vi "Get All.vi"(0 "Tree Reference In":refnum<vi>, 2 "Starting Tag":string, 3 "Input Tree Items(DO NOT WIRE)":string[](array[string]), 5 "error in (no error)":errorcluster) -> (14 "Tree Reference Out":refnum<vi>, 16 "Current Item":string, 17 "Output Tree Items":string[](array[string]), 19 "error out":errorcluster)   [LabVIEW 2011, in "VITesterUtilities.lvlib"]
doc: "Retrieves all elements in tree at and below the starting tag. When Starting Tag and Input Tree Items are left unwired it will return all elements in the tree."
uses:
  Libraries/VITesterUtilities.lvlib
panel:
  in  "Identical VI Refnum":refnum<vi>
  # "VI LOCALS"
  # "VI OUTPUTS"
  # "VI INPUTS"
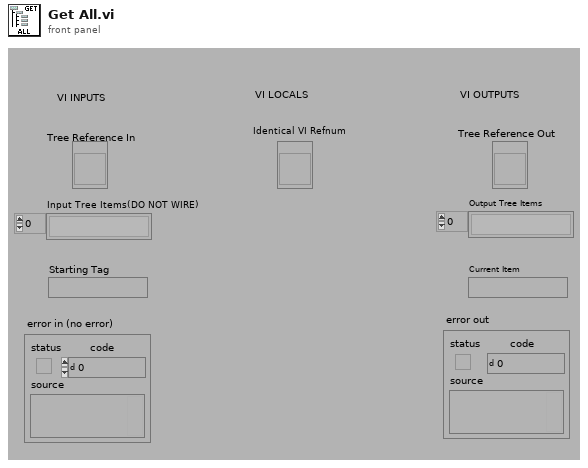
[diagram p1: front panel]
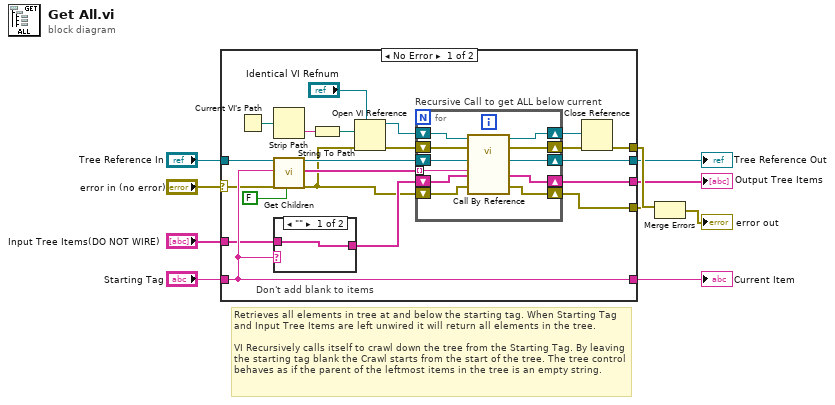
[diagram p0: block diagram]
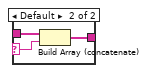
[diagram p2: hidden frame]
diagram:
  # "Retrieves all elements in tree at and below the starting tag. When Starting Tag and Input Tree Items are left unwired it will return all elements in the tree. \n\nVI Recursively calls itself to crawl down the tree from the Starting Tag. By leaving the starting tag blank the Crawl starts from the start of the tree. The tree control behaves as if the parent of the leftmost items in the tree is an empty string."
  n1 = case shown="No Error" "error in (no error)" {
    selector: "error in (no error)" -> [w12 w47]
    tunnel: "Tree Reference In" -> [w31 w48]
    tunnel: [w30 w48] -> w6
    tunnel: "Starting Tag" -> [w29 w50]
    tunnel: [w28 w49] -> w4
    tunnel: [w29 w50] -> w3
    tunnel: "Input Tree Items(DO NOT WIRE)" -> [w27 w49]
    tunnel: [w26 w47] -> w10
    tunnel: [w25 w47] -> w9
    frame No Error {
      n2 = Current VI's Path() -> (path=w17:path)
      n3 = Strip Path(path=w17) -> (name=w15:string)  [unwired: 1 out]
      n4 = call "Get Children.vi"("Tree Reference In"=w31, "Parent Tag"=w29, "error in (no error)"=w12, "Use Current"=FALSE) -> ("Tree Reference Out"=w24:refnum<vi>, "Children Tags"=w20:string[], "error out"=w11:errorcluster)  [unwired: 13 in]
      n5 = case "Don't add blank to items" shown="\"\"" w29 {
        selector: w29 -> [_ w33]
        tunnel: w27 -> [w32 w35]
        tunnel: [w32 w34] -> w19
        frame "" {
        }
        frame Default {
          n6 = Build Array (concatenate)(w35, w33) -> (w34:string[])
        }
      }
      n7 = String To Path(string=w15) -> (path=w16:path)
      n8 = Open VI Reference(type specifier VI Refnum (for type only)="Identical VI Refnum", vi path=w16, error in (no error)=w11) -> (vi reference=w18:refnum<vi>, error out=w22:errorcluster)  [unwired: 3 in]
      n9 = for "Recursive Call to get ALL below current" {
        shift-right: [w44] -> w25
        shift-left: w11 -> [w45]
        shift-right: [w43] -> w30
        shift-left: w24 -> [w46]
        shift-right: [w40] -> w21
        shift-left: w22 -> [w41]
        shift-right: [w36] -> w23
        shift-left: w18 -> [w42]
        tunnel: w20 -> [w39] mode=indexing
        shift-right: [w38] -> w28
        shift-left: w19 -> [w37]
        n10 = call-by-ref "?"(reference=w42, error in=w41, "Tree Reference In"=w46, "Starting Tag"=w39, "Input Tree Items(DO NOT WIRE)"=w37, "error in (no error)"=w45) -> (reference out=w36:refnum<vi>, error out=w40:errorcluster, "Tree Reference Out"=w43:refnum<vi>, "Output Tree Items"=w38:string[], 19:"error out"=w44:errorcluster)  [unwired: 12 in, 1 out]
      }
      n11 = Close Reference(reference=w23, error in (no error)=w21) -> (error out=w26:errorcluster)
    }
    frame Error {
    }
  }
  "Tree Reference Out" <- w6
  "Output Tree Items" <- w4
  "Current Item" <- w3
  n12 = Merge Errors(w10, w9) -> (→"error out":errorcluster)
